vi "MultiplyOrDontX0.vi"(9 "Numeric 3":i32, 10 "Numeric 4":i32, 11 "Numeric in":dbl) -> (3 "Numeric out":dbl)   [LabVIEW 2014]
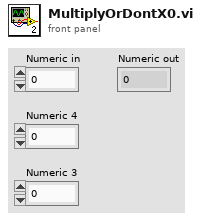
[diagram p1: front panel]
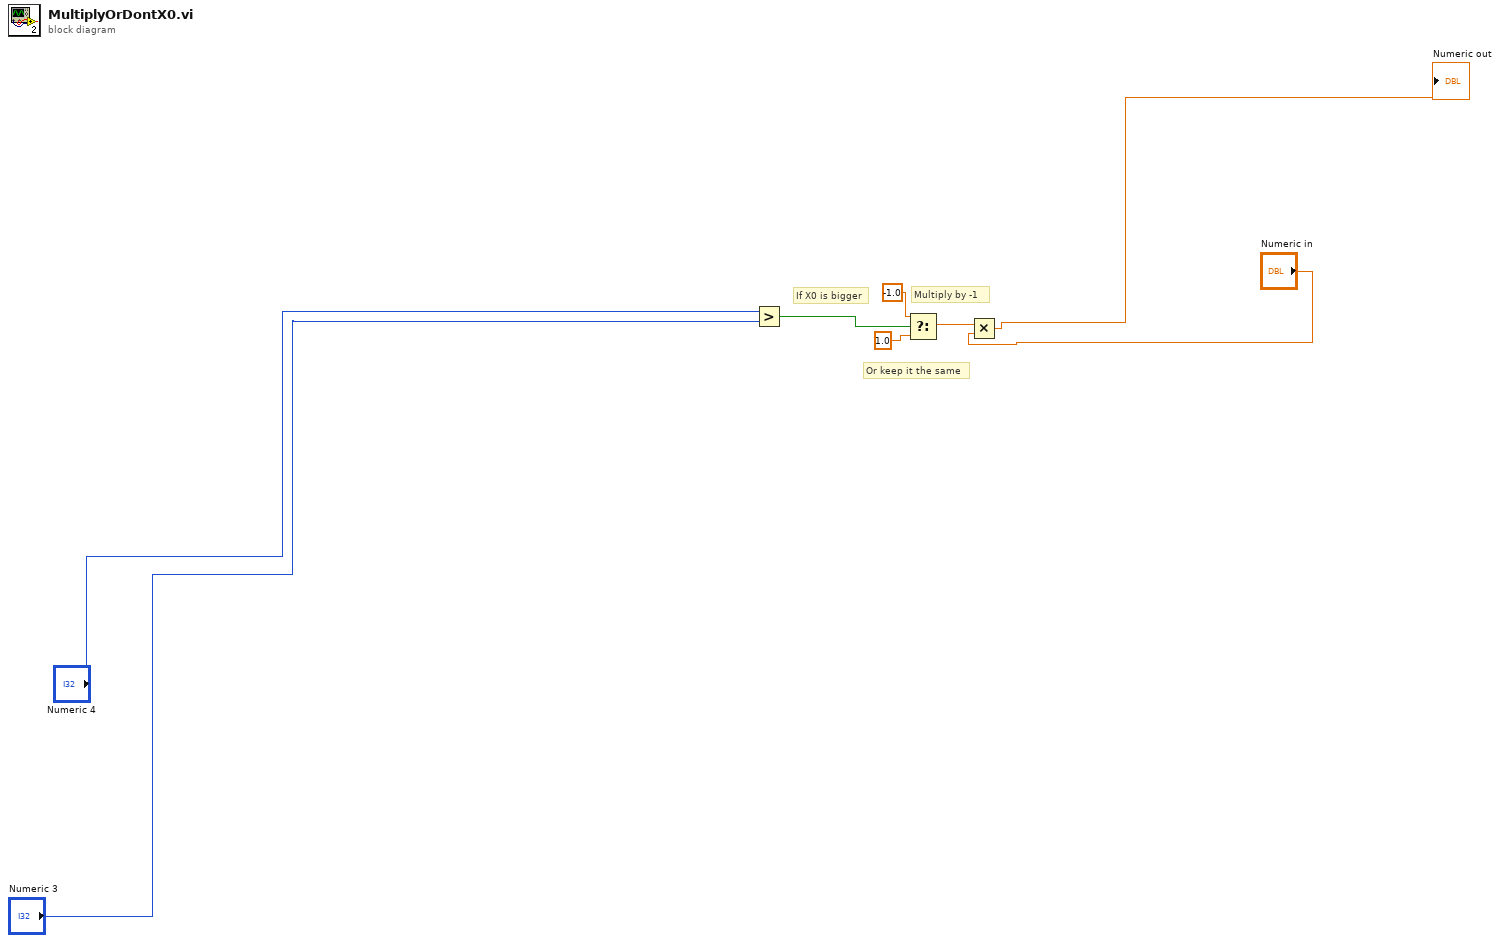
[diagram p0: block diagram]
diagram:
  # "Or keep it the same"
  # "Multiply by -1"
  # "If X0 is bigger"
  n1 = Greater?(x="Numeric 4", y="Numeric 3") -> (0:w3:bool)
  n2 = Select(t=-1.0, s=w3, f=1.0) -> (s? t:f=w6:dbl)
  n3 = Multiply(x=w6, y="Numeric in") -> (x*y=→"Numeric out":dbl)
